vi "spectrum_suavization.vi"(9 "order":i32=4, 10 "freq":dbl=0.4 format="%#_13g", 11 "data":cluster{"freqs":dbl[], "Array":dbl[]}) -> (2 "freqs":dbl[](array[numeric]), 3 "ampltiude":dbl[](array[numeric]))   [LabVIEW 2018]
uses:
  <vilib>/Analysis/3filter.llb/Filter Passband Type.ctl
  <vilib>/Analysis/3filter.llb/Butterworth Filter (DBL).vi
  <vilib>/Analysis/NI_AALBase.lvlib
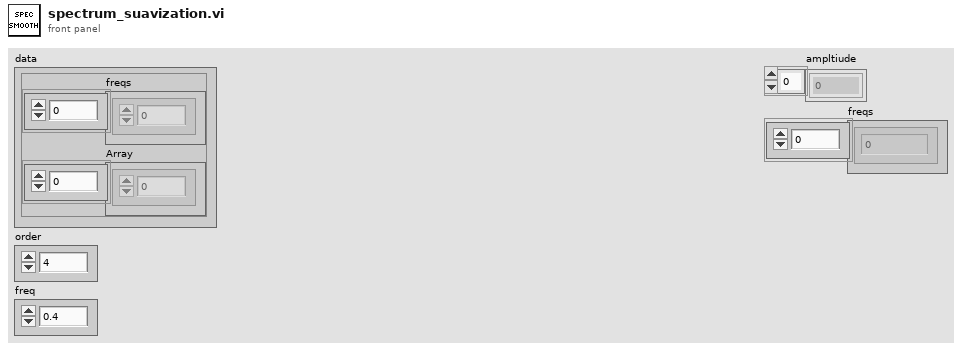
[diagram p1: front panel]
types:
  T1 = typedef "NI_AALBase.lvlib/Filter Passband Type.ctl" = enum32{"Lowpass", "Highpass", "Bandpass", "Bandstop"}
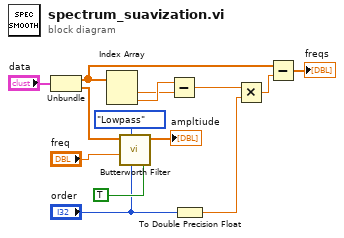
[diagram p0: block diagram]
diagram:
  n1 = Unbundle("data") -> ("freqs"=w4:dbl[], "Array"=w10:dbl[])
  n2 = Index Array(array=w4) -> (element #1=w13:dbl, element #2=w14:dbl)  [unwired: 2 in]
  n3 = call-poly <vilib>:"Butterworth Filter.vi"("init/cont (init:F)"=TRUE, "order"="order", "filter type"=Filter_Passband_Type."Lowpass", "high cutoff freq: fh"="freq", "X"=w10) -> ("Filtered X"=→"ampltiude":dbl[])  [unwired: 3 in, 1 out]
  n4 = Subtract(x=w14, y=w13) -> (x-y=w6:dbl)
  n5 = To Double Precision Float(number="order") -> (double precision float=w5:dbl)
  n6 = Multiply(x=w6, y=w5) -> (x*y=w3:dbl)
  n7 = Subtract(x=w4, y=w3) -> (x-y=→"freqs":dbl[])
